vi "Modules Selector.vi"(10 "Modules Types In":T2[](array[typedef]), 11 "DQMH Modules In":refnum<vi>[](array[refnum])) -> (1 "Descriptions":string[](array[string]), 2 "Modules Types Out":T2[](array[typedef]), 3 "DQMH Modules Out":refnum<vi>[](array[refnum]))   [LabVIEW 2023, in "Panther Dashboard.lvlib"]
uses:
  Panther Dashboard.lvlib
  Module type--enum.ctl
  Module to scan--cluster.ctl
panel:
  in  "DQMH Modules found in Project":T1[](array[typedef])
  in  "Scan Selection":bool
  in  "Select/Unselect All":bool
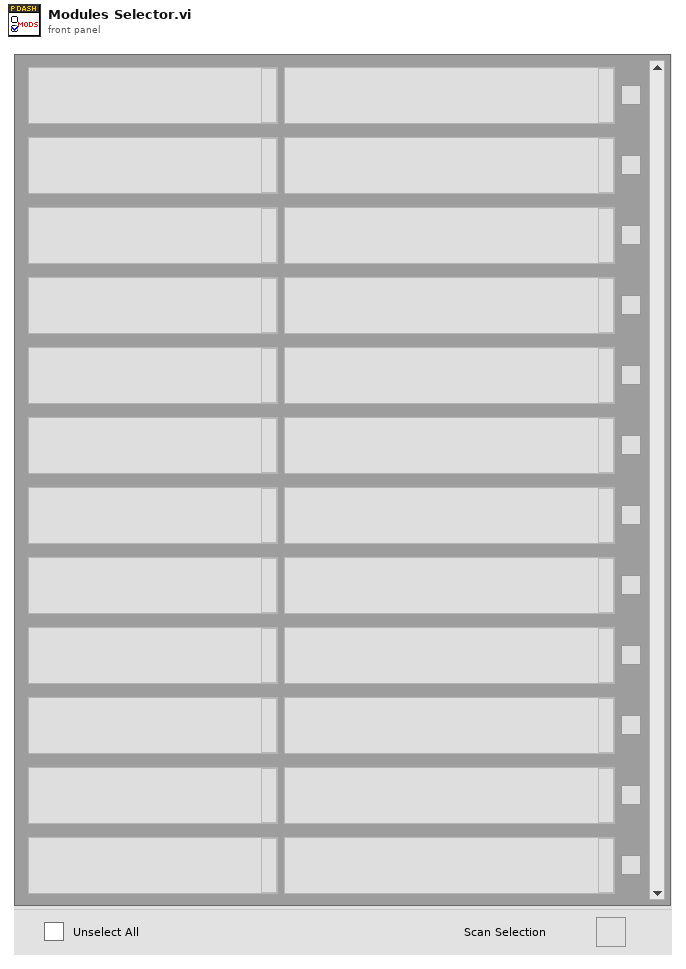
[diagram p1: front panel]
types:
  T1 = typedef "Panther Dashboard.lvlib/Module to scan--cluster.ctl" = cluster{"Module Name":string, "Description":string, "Scan?":bool}
  T2 = typedef "Panther Dashboard.lvlib/Module type--enum.ctl" = enum16{"Module type: Singleton", "Module type: Cloneable"}
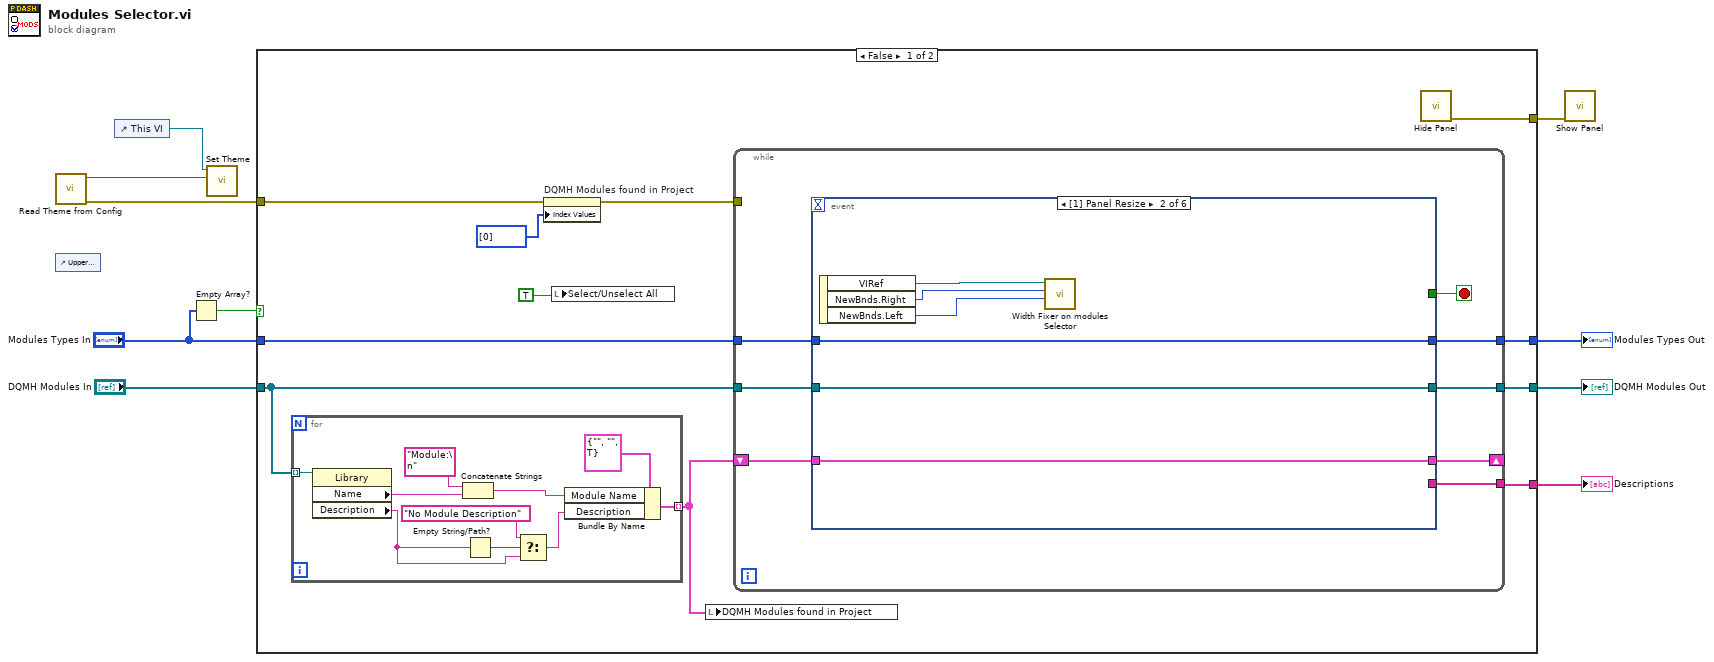
[diagram p0: block diagram]
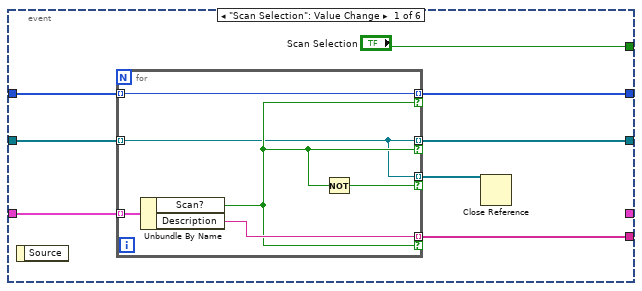
[diagram p2: hidden frame]
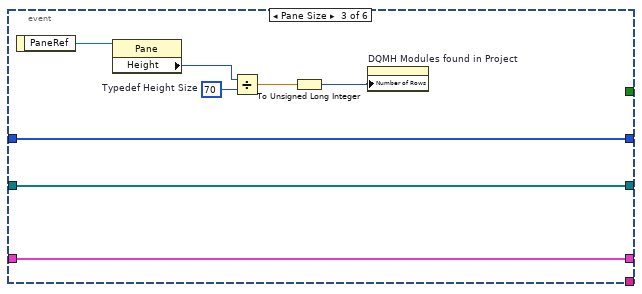
[diagram p3: hidden frame]
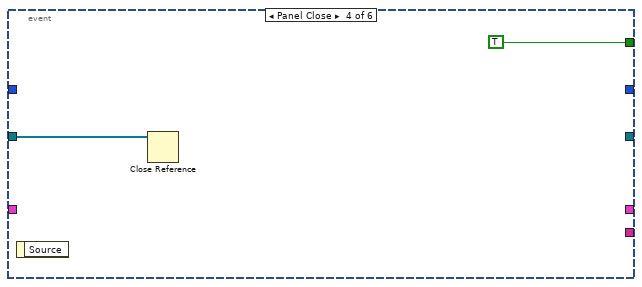
[diagram p4: hidden frame]
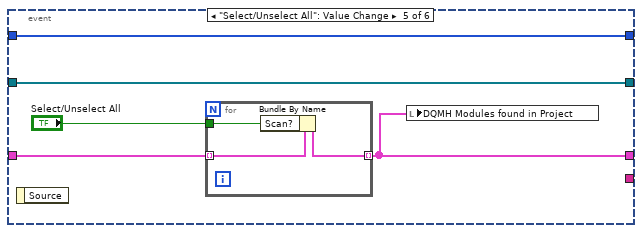
[diagram p5: hidden frame]
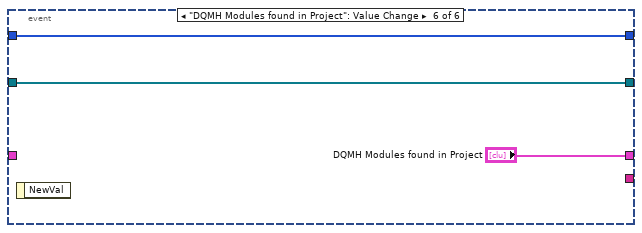
[diagram p6: hidden frame]
diagram:
  n1 = call "Read Theme from Config.vi"() -> ("error out"=w10:errorcluster, "Theme"=w4:bool)  [unwired: 10 in]
  n2 = control-ref of="Upper Pane"() -> ()  [unwired: 1 out]
  n3 = control-ref of="This VI"() -> (w5:refnum<vi>)
  n4 = Empty Array?(array="Modules Types In") -> (empty?=w2:bool)
  n5 = call "Set Theme.vi"("Dark?"=w4, "VI in"=w5) -> ()  [unwired: 10 in]
  n6 = case shown="False" w2 {
    tunnel: "DQMH Modules In" -> [w14 _]
    tunnel: [w18 _] -> w1
    tunnel: "Modules Types In" -> [w17 _]
    tunnel: [w16 _] -> w7
    tunnel: [w15 _] -> w6
    tunnel: w10 -> [w20 _]
    tunnel: [w21 _] -> w9
    frame False {
      n7 = for {
        tunnel: w14 -> [w31] mode=indexing
        tunnel: [w30] -> w13 mode=indexing
        n8 = property class="Library"(reference=w31) -> ("Name"=w28:string, "Description"=w26:string)  [unwired: 1 in, 2 out]
        n9 = Concatenate Strings("Module:\n" ("string"), w28) -> (w23:string)
        n10 = Empty String/Path?(string/path=w26) -> (empty?=w27:bool)
        n11 = Select(t="No Module Description", s=w27, f=w26) -> (s? t:f=w25:string)
        n12 = Bundle By Name(cluster=T1 {"Module Name"="", "Description"="", "Scan?"=TRUE} ("Module"), "Module Name"=w23, "Description"=w25) -> (w30:T1)
      }
      n13 = property on="DQMH Modules found in Project" class="Arr (strict)"(error in=w20, "Index Values"=u32[] [0]) -> (error out=w19:errorcluster)  [unwired: 1 in, 1 out]
      n14 = local write "Select/Unselect All"(TRUE ("Select /Unselect All Modules")) -> ()
      n15 = local write "DQMH Modules found in Project"(w13) -> ()
      n16 = while {
        shift-right: [w37] -> _
        shift-left: w13 -> [w39]
        tunnel: w14 -> [w36]
        tunnel: [w35] -> w18
        tunnel: w17 -> [w34]
        tunnel: [w33] -> w16
        tunnel: [w32] -> w15
        tunnel: w19 -> [_]
        stop <- w38 stop-if-true
        n17 = event shown="[1] Panel Resize" {
          selector: _ -> [_ _ _ _ _ _]
          dyn-events: _ -> [_ _ _ _ _ _]
          timeout: _ -> [_ _ _ _ _ _]
          tunnel: w39 -> [w47 w57 w63 _ w72 _]
          tunnel: ["Scan Selection" _ _ TRUE ("All") _ _] -> w38
          tunnel: [_ w57 w63 _ w71 "DQMH Modules found in Project"] -> w37
          tunnel: [w43 w58 w61 _ w73 w80] -> w35
          tunnel: w36 -> [w45 w58 w61 w68 w73 w80]
          tunnel: w34 -> [w46 w59 w62 _ w74 w79]
          tunnel: [w44 w59 w62 _ w74 w79] -> w33
          tunnel: [w42 _ _ _ _ _] -> w32
          event "Scan Selection": Value Change {
            n18 = event-data() -> ()  [unwired: 1 in, 1 out]
            n19 = for {
              tunnel: w47 -> [w53] mode=indexing
              tunnel: [w52] -> w42 mode=indexing if=w50
              tunnel: w46 -> [w51] mode=indexing
              tunnel: w45 -> [w49] mode=indexing
              tunnel: [w51] -> w44 mode=indexing if=w50
              tunnel: [w49] -> w43 mode=indexing if=w50
              tunnel: [w49] -> w41 mode=indexing if=w48
              n20 = Unbundle By Name(w53) -> ("Scan?"=w50:bool, "Description"=w52:string)
              n21 = Not(x=w50) -> (.not. x?=w48:bool)
            }
            n22 = Close Reference(reference=w41) -> ()  [unwired: 1 in, 1 out]
          }
          event Panel Resize {
            n23 = event-data() -> ("VIRef"=w56:refnum<vi>, "NewBnds.Right"=w54:i16, "NewBnds.Left"=w55:i16)  [unwired: 1 in]
            n24 = call "Width Fixer on modules Selector.vi"("Left"=w55, "Right"=w54, "VI in"=w56) -> ()  [unwired: 9 in]
          }
          event Pane Size {
            w65 = u32 70  # Typedef Height Size
            n25 = event-data() -> ("PaneRef"=w67:refnum<vi>)  [unwired: 1 in]
            n26 = property class="Pane"(reference=w67) -> ("Height"=w66:u32)  [unwired: 1 in, 2 out]
            n27 = Divide(x=w66, y=w65) -> (x/y=w64:dbl)
            n28 = To Unsigned Long Integer(number=w64) -> (unsigned 32bit integer=w60:u32)
            n29 = property on="DQMH Modules found in Project" class="Arr (strict)"("Number of Rows"=w60) -> ()  [unwired: 2 in, 2 out]
          }
          event Panel Close {
            n30 = event-data() -> ()  [unwired: 1 in, 1 out]
            n31 = Close Reference(reference=w68) -> ()  [unwired: 1 in, 1 out]
          }
          event "Select/Unselect All": Value Change {
            n32 = event-data() -> ()  [unwired: 1 in, 1 out]
            n33 = for {
              tunnel: w72 -> [w77] mode=indexing
              tunnel: [w76] -> w71 mode=indexing
              tunnel: "Select/Unselect All" -> [w75]
              n34 = Bundle By Name(cluster=w77, "Scan?"=w75) -> (w76:T1)
            }
            n35 = local write "DQMH Modules found in Project"(w71) -> ()
          }
          event "DQMH Modules found in Project": Value Change {
            n36 = event-data() -> ()  [unwired: 1 in, 1 out]
          }
        }
      }
      n37 = call "Hide Panel.vi"() -> ("error out"=w21:errorcluster)  [unwired: 11 in]
    }
    frame True {
    }
  }
  "Modules Types Out" <- w7
  "DQMH Modules Out" <- w1
  "Descriptions" <- w6
  n38 = call "Show Panel.vi"("error in (no error)"=w9) -> ()  [unwired: 10 in, 1 out]
